vi "Is VI Server Required.vi"(8 "error in (no error)":errorcluster, 11 "Keyboard Action in":refnum<class "Keyboard Action.lvclass">) -> (0 "error out":errorcluster, 2 "VI Server Required?":bool, 3 "Keyboard Action out":refnum<class "Keyboard Action.lvclass">)   [LabVIEW 2020, in "MacroAssert.lvlib" / "Keyboard Action.lvclass"]
doc: "Outputs whether VI Server is required to perform the given step."
uses:
  Keyboard Action.lvclass
  Keyboard Action.lvclass/Keyboard Action.ctl
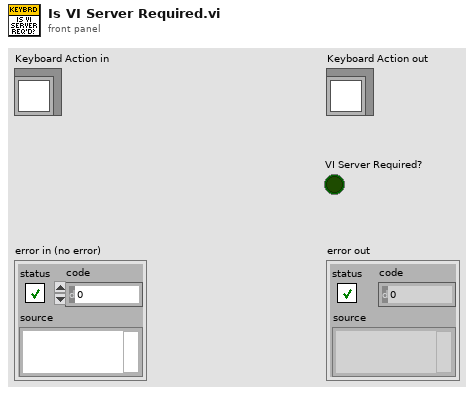
[diagram p1: front panel]
types:
  T1 = typedef "MacroAssert.lvlib/Keyboard Action.lvclass/Keyboard Action Type.ctl" = enum16{"Key Press", "Key Down", "Key Up", "Key Sequence"}
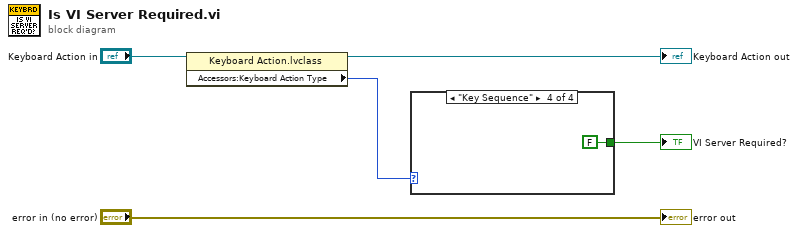
[diagram p0: block diagram]
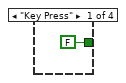
[diagram p2: hidden frame]
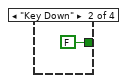
[diagram p3: hidden frame]
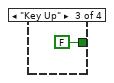
[diagram p4: hidden frame]
diagram:
  n1 = property class="Keyboard Action.lvclass"(reference="Keyboard Action in") -> (reference out=→"Keyboard Action out":refnum<class "Keyboard Action.lvclass">, "Accessors:Keyboard Action Type"=w4:T1)  [unwired: 1 in, 1 out]
  n2 = case shown="\"Key Sequence\"" w4 {
    tunnel: [FALSE FALSE FALSE FALSE] -> w2
    frame "Key Press" {
    }
    frame "Key Down" {
    }
    frame "Key Up" {
    }
    frame "Key Sequence" {
    }
  }
  "VI Server Required?" <- w2
  "error out" <- "error in (no error)"
